vi "getStartTrigger.vi"(8 "error in (no error)":errorcluster, 11 "CameraManager in":refnum<class "CameraManager.lvclass">) -> (0 "error out":errorcluster, 2 "start_trigger":string, 3 "CameraManager out":refnum<class "CameraManager.lvclass">)   [LabVIEW 2011, in "iManagement.lvlib" / "CameraManager.lvclass"]
uses:
  CameraManager.lvclass
  CameraManager.lvclass/CameraManager.ctl
  Hal/Channels/Camera/CameraController.lvclass
  Hal/Channels/Camera/CameraEventsManager/CameraEventsManger.lvclass
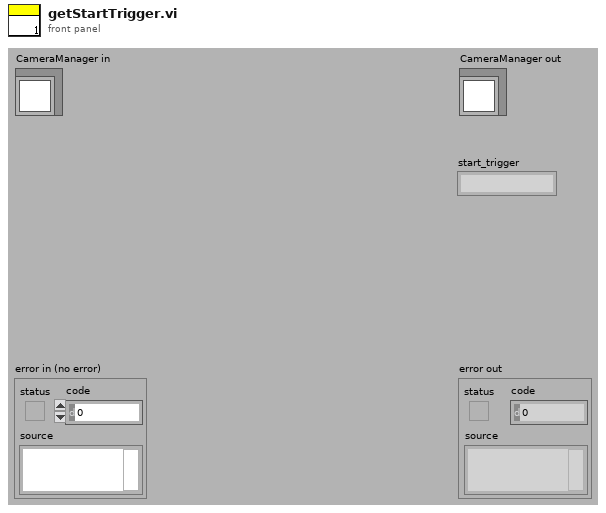
[diagram p1: front panel]
types:
  T1 = enum16{"Number", "String", "NumberArray", "StringArray", "xmlNode"}
  T2 = cluster{"settingsFrontEndEvents":cluster{"loadSettingsFromPath":refnum<user-event>, "lookUpElementEvent":refnum<user-event>, "saveSettings":refnum<user-event>, "loadSettings":refnum<user-event>, "close":refnum<user-event>, "replaceElement":refnum<user-event>, "findParentNodes":refnum<user-event>, "createNode":refnum<user-event>}, "settingBackEndEvents":cluster{"defaultSettingsPathRequest":refnum<user-event>, "searchResultEvent":refnum<user-event>, "settingsSaved":refnum<user-event>, "settingsLoaded":refnum<user-event>, "foundParentNode":refnum<user-event>}}
  T3 = cluster{"lookUpElement":string, string, "typeEnum":enum16{"Number", "String", "NumberArray", "StringArray", "xmlNode"}}
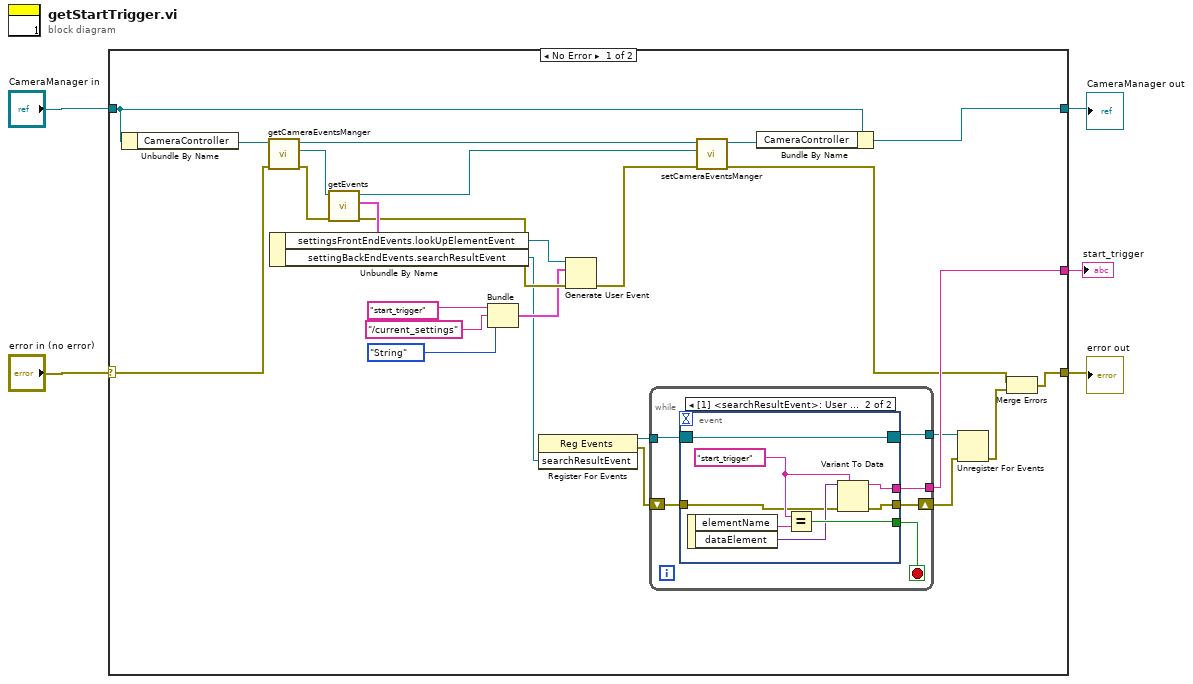
[diagram p0: block diagram]
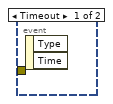
[diagram p2: hidden frame]
diagram:
  n1 = case shown="No Error" "error in (no error)" {
    selector: "error in (no error)" -> [w22 w47]
    tunnel: [w7 w47] -> w4
    tunnel: [w16 w46] -> w2
    tunnel: "CameraManager in" -> [w17 w46]
    tunnel: [w11 _] -> w1
    frame No Error {
      n2 = Unbundle By Name(w17) -> ("CameraController"=w29:refnum<class "CameraController.lvclass">)
      n3 = call-dynamic "getCameraEventsManger.vi"("error in (no error)"=w22, "CameraController.lvclass in"=w29) -> ("error out"=w30:errorcluster, "Hardware:Channels.lvlib:CameraEventsManger.lvclass"=w31:refnum<class "CameraEventsManger.lvclass">, "CameraController.lvclass out"=w28:refnum<class "CameraController.lvclass">)  [unwired: 7 in]
      n4 = call-dynamic "getEvents.vi"("error in (no error)"=w30, "CameraEventsManger in"=w31) -> ("error out"=w24:errorcluster, "settingsEvents"=w25:T2, "CameraEventsManger out"=w26:refnum<class "CameraEventsManger.lvclass">)  [unwired: 5 in, 2 out]
      n5 = Unbundle By Name(w25) -> ("settingsFrontEndEvents.lookUpElementEvent"=w15:refnum<user-event>, "settingBackEndEvents.searchResultEvent"=w13:refnum<user-event>)
      n6 = Bundle("lookUpElement"="start_trigger", "/current_settings", "typeEnum"=T1."String") -> (w18:T3)  [unwired: 1 in]
      n7 = register-events(w13) -> (reference out=w14:refnum<event-registration>, error out=w12:errorcluster)  [unwired: 2 in]
      n8 = Generate User Event(user event=w15, event data cluster=w18, error in=w24) -> (error out=w23:errorcluster)  [unwired: 1 out]
      n9 = while {
        tunnel: w14 -> [w37]
        shift-right: [w34] -> w9
        shift-left: w12 -> [w35]
        tunnel: [w33] -> w11
        tunnel: [w32] -> w10
        stop <- w36 stop-if-true
        n10 = event shown="[1] <searchResultEvent>: User Event" {
          selector: w37 -> [_ w38]
          dyn-events: [_ w38] -> w32
          timeout: _ -> [_ _]
          tunnel: [_ w45] -> w36
          tunnel: w35 -> [_ w41]
          tunnel: [_ w40] -> w34
          tunnel: [_ w39] -> w33
          event Timeout {
            n11 = event-data() -> ()  [unwired: 1 in, 2 out]
          }
          event User Event {
            w43 = "start_trigger" ("lookUpElement")
            n12 = event-data() -> ("elementName"=w44:string, "dataElement"=w42:variant)  [unwired: 1 in]
            n13 = Equal?(x=w43, y=w44) -> (x = y?=w45:bool)
            n14 = Variant To Data(error in=w41, type=w43, Variant=w42) -> (data=w39:string, error out=w40:errorcluster)
          }
        }
      }
      n15 = call-dynamic "setCameraEventsManger.vi"("error in (no error)"=w23, "Hardware:Channels.lvlib:CameraEventsManger.lvclass"=w26, "CameraController.lvclass in"=w28) -> ("error out"=w8:errorcluster, "CameraController.lvclass out"=w27:refnum<class "CameraController.lvclass">)  [unwired: 7 in]
      n16 = Bundle By Name(cluster=w17, "CameraController"=w27) -> (w16:refnum<class "CameraManager.lvclass">)
      n17 = Unregister For Events(event registration refnum=w10, error in=w9) -> (error out=w6:errorcluster)
      n18 = Merge Errors(w8, w6) -> (w7:errorcluster)
    }
    frame Error {
    }
  }
  "error out" <- w4
  "CameraManager out" <- w2
  "start_trigger" <- w1
